vi "Extract Section End Points.vi"(0 "Section Range":string) -> (1 "Section End Points":i32[](array[numeric]), 2 "Section End":i32, 3 "Section Start":i32)   [LabVIEW 2020, in "AoC 2022.lvlib"]
uses:
  AoC 2022.lvlib
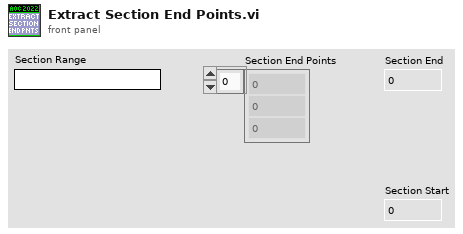
[diagram p1: front panel]
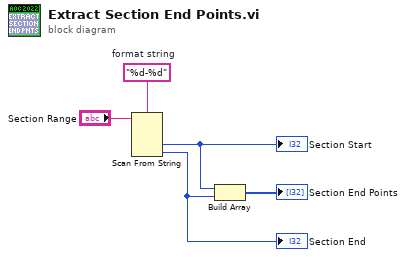
[diagram p0: block diagram]
diagram:
  w4 = "%d-%d"  # format string
  n1 = Scan From String(format string=w4, input string="Section Range") -> (output 1=w3:i32, output 2=w2:i32)  [unwired: 4 in, 3 out]
  "Section Start" <- w3
  "Section End" <- w2
  n2 = Build Array(w3, w2) -> (→"Section End Points":i32[])
